vi "Enforce N Button Switch.vi"(8 "error in (no error)":errorcluster, 10 "banner gui refs":T1[](array[typedef]), 11 "boolean reference in":refnum<vi>) -> (0 "error out":errorcluster, 3 "selected gui pairing":T1)   [LabVIEW 2020]
uses:
  GUI References.ctl
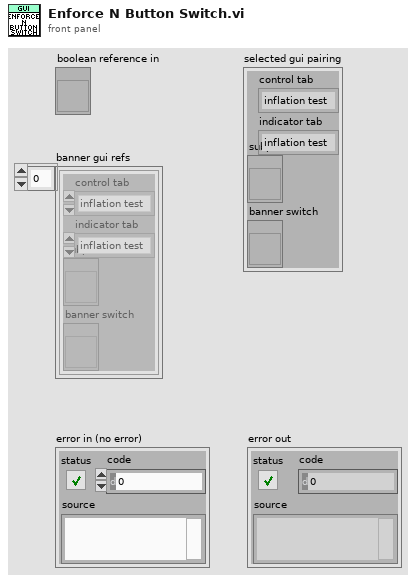
[diagram p1: front panel]
types:
  T1 = typedef "GUI References.ctl" = cluster{"control tab":enum32{"inflation test", "force calibration", "camera calibration", "test equipment"}, "indicator tab":enum32{"inflation test", "force calibration", "camera calibration", "test equipment"}, "subpanel vi":refnum<vi>, "banner switch":refnum<vi>}
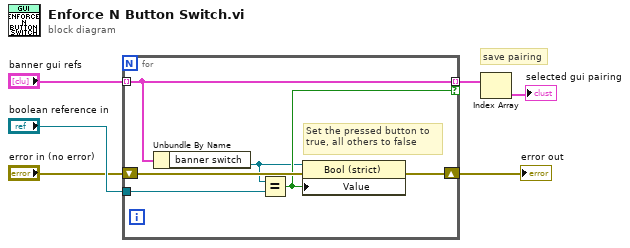
[diagram p0: block diagram]
diagram:
  # "save pairing"
  n1 = for {
    shift-right: [w10] -> w5
    shift-left: "error in (no error)" -> [w11]
    tunnel: "boolean reference in" -> [w12]
    tunnel: [w7] -> w3 mode=indexing if=w9
    tunnel: "banner gui refs" -> [w7] mode=indexing
    # "Set the pressed button to true, all others to false"
    n2 = Unbundle By Name(w7) -> ("banner switch"=w8:refnum<vi>)
    n3 = Equal?(x=w8, y=w12) -> (x = y?=w9:bool)
    n4 = property class="Bool (strict)"(reference=w8, error in=w11, "Value"=w9) -> (error out=w10:errorcluster)  [unwired: 1 out]
  }
  "error out" <- w5
  n5 = Index Array(array=w3) -> (element=→"selected gui pairing":T1)  [unwired: 1 in]
